vi "CL_Format PID Parameters.vi"(0 "PID Cfg":dbl[](array[numeric]) format="%.2f", 9 "PID gain schedule":T1(array[cluster])=[{"PID gains"={"proportional gain (Kc)"=1.0, "integral time (Ti, min)"=0.01, "derivative time (Td, min)"=0.0}, "max value"=100.0}] {"max value" format="%.2f"; "PID gains"."derivative time (Td, min)" format="%.3f"; "PID gains"."integral time (Ti, min)" format="%.3f"; "PID gains"."proportional gain (Kc)" format="%.3f"}, 11 "error in":errorcluster) -> (1 "Manual":dbl format="%.2f", 2 "Mode":bool caption="True:Auto\nFalse:Manual", 3 "output range":cluster{"output high":dbl, "output low":dbl}={"output high"=100.0, "output low"=-100.0} {"output low" format="%.2f"; "output high" format="%.2f"}, 4 "Setpoint":dbl format="%.2f", 6 "Process Variable":dbl format="%.2f", 10 "PID gains out":T2={"proportional gain (Kc)"=1.0, "integral time (Ti, min)"=0.01, "derivative time (Td, min)"=0.0} {"derivative time (Td, min)" format="%.3f"; "integral time (Ti, min)" format="%.3f"; "proportional gain (Kc)" format="%.3f"}, 14 "Gain Schedule Variable":dbl format="%.2f", 15 "error out":errorcluster)   [LabVIEW 2010]
doc: "Parses PID parameter array into data types for NI Array based PID VI.\n\n2007 Mike Ashe\nmichael.ashe@imaginatics.net\nCell: 860-961-0876"
uses:
  <vilib>/addons/control/pid/pid.llb/PID Gain Schedule (DBL).vi
  <vilib>/addons/control/pid/NI_PID_pid.lvlib
panel:
  out "Reinit (Not used)":bool
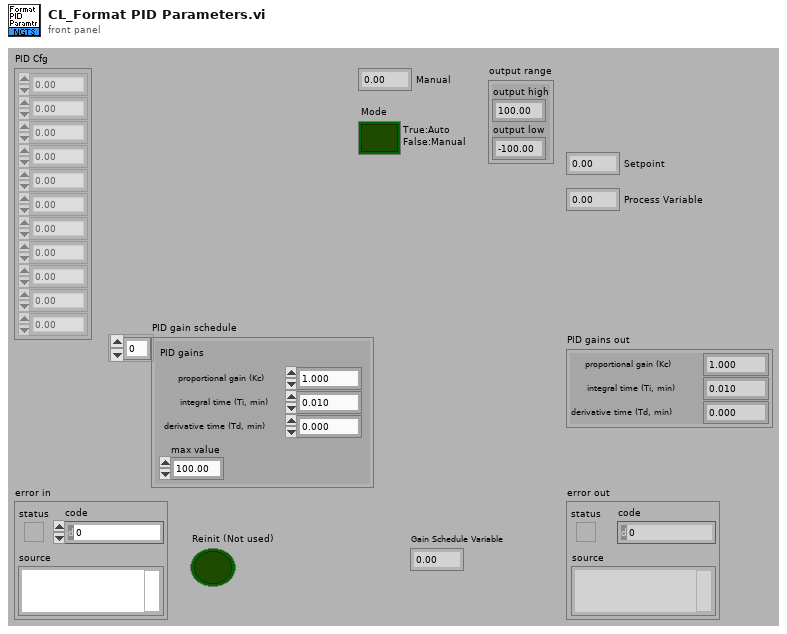
[diagram p1: front panel]
types:
  T1 = cluster{"PID gains":cluster{"proportional gain (Kc)":dbl, "integral time (Ti, min)":dbl, "derivative time (Td, min)":dbl}, "max value":dbl}[]
  T2 = cluster{"proportional gain (Kc)":dbl, "integral time (Ti, min)":dbl, "derivative time (Td, min)":dbl}
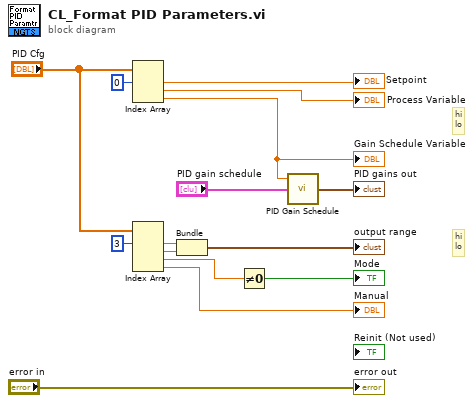
[diagram p0: block diagram]
diagram:
  # "hi\nlo"
  # "hi\nlo"
  n1 = Index Array(array="PID Cfg", index #1=0 ("index")) -> (element #1=→"Setpoint":dbl, element #2=→"Process Variable":dbl, element #3=w1:dbl)  [unwired: 2 in]
  "Gain Schedule Variable" <- w1
  n2 = Index Array(array="PID Cfg", index #1=3 ("index")) -> (element #1=w6:dbl, element #2=w7:dbl, element #3=w4:dbl, element #4=→"Manual":dbl)  [unwired: 3 in]
  n3 = Bundle("Numeric"=w6, "Numeric"=w7) -> (→"output range":cluster{"Numeric":dbl, "Numeric":dbl})  [unwired: 1 in]
  n4 = Not Equal To 0?(x=w4) -> (x != 0?=→"Mode":bool)
  n5 = call-poly <vilib>:"PID Gain Schedule.vi"("PID gain schedule"="PID gain schedule", "gain scheduling value"=w1) -> ("PID gains out"=→"PID gains out":T2)  [unwired: 2 in, 1 out]
  "error out" <- "error in"
